vi "Java_Util.vi"(10 "Limit":dbl format="%#_13g", 11 "V":dbl format="%#_13g") -> (3 "V Out":dbl)   [LabVIEW 2017]
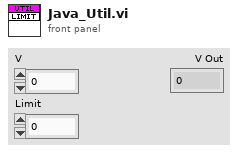
[diagram p1: front panel]
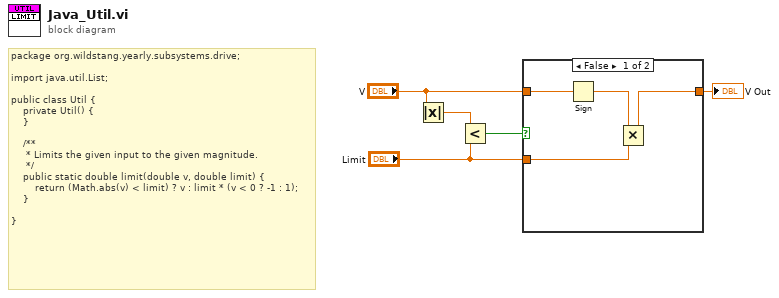
[diagram p0: block diagram]
diagram:
  # "package org.wildstang.yearly.subsystems.drive;\n\nimport java.util.List;\n\npublic class Util {\n    private Util() {\n    }\n\n    /**\n     * Limits the given input to the given magnitude.\n     */\n    public static double limit(double v, double limit) {\n        return (Math.abs(v) < limit) ? v : limit * (v < 0 ? -1 : 1);\n    }\n\n}"
  n1 = Absolute Value(x="V") -> (abs(x)=w5:dbl)
  n2 = Less?(x=w5, y="Limit") -> (x < y?=w4:bool)
  n3 = case shown="False" w4 {
    tunnel: "V" -> [w9 w10]
    tunnel: [w6 w10] -> w2
    tunnel: "Limit" -> [w7 _]
    frame False {
      n4 = Sign(1:w9) -> (0:w8:dbl)
      n5 = Multiply(x=w8, y=w7) -> (x*y=w6:dbl)
    }
    frame True {
    }
  }
  "V Out" <- w2
